vi "Winch Global.vi"() -> ()   [LabVIEW 2016]
panel:
  out "Winch Moving":bool
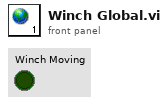
[diagram p1: front panel]
diagram:
